vi "Available Data.vi"(8 "error in (no error)":errorcluster, 11 "Picam in":refnum<class "Picam.lvclass">) -> (0 "error out":errorcluster, 1 "Running?":bool, 2 "Data Available?":bool, 3 "Picam out":refnum<class "Picam.lvclass">)   [LabVIEW 2019, in "Picam.lvclass"]
uses:
  Picam.lvclass
  Picam.lvclass/Picam.ctl
  picam32_LabView_SDK/PICam_lib/PICam.lvlib
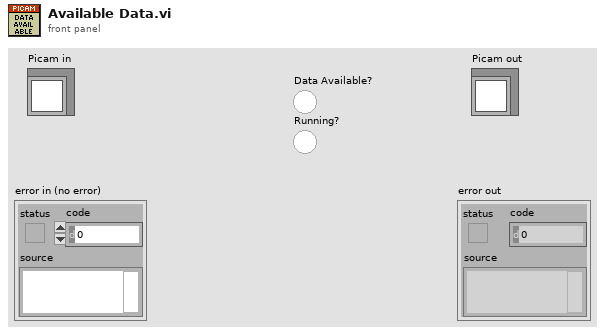
[diagram p1: front panel]
types:
  T1 = typedef "PICam.lvlib/PicamAcquisitionStatus.ctl" = cluster{"running":i32, "errors":T2, "readout_rate":dbl}
  T2 = typedef "PICam.lvlib/PicamAcquisitionErrorsMask.ctl" = enum8{"None", "DataLost", "ConnectionLost", "3", "DataNotArriving", "5", "6", "7", "ShutterOverheated", "9", "10", "11", "12", "13", "14", "15", "CameraFaulted"}
  T3 = typedef "PICam.lvlib/PicamAvailableData.ctl" = cluster{"initial_readout":u64, "readout_count":i64}
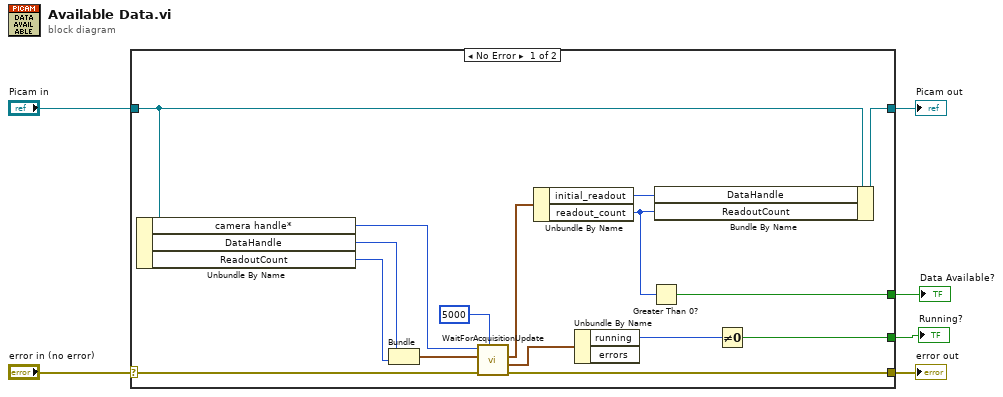
[diagram p0: block diagram]
diagram:
  n1 = case shown="No Error" "error in (no error)" {
    selector: "error in (no error)" -> [w22 w24]
    tunnel: [w20 w24] -> w5
    tunnel: [w16 w23] -> w3
    tunnel: "Picam in" -> [w21 w23]
    tunnel: [w17 _] -> w2
    tunnel: [w11 _] -> w1
    frame No Error {
      n2 = Unbundle By Name(w21) -> ("camera handle*"=w19:u64, "DataHandle"=w8:u64, "ReadoutCount"=w7:i64)
      n3 = Bundle("DataHandle"=w8, "ReadoutCount"=w7) -> (w9:cluster{"DataHandle":u64, "ReadoutCount":i64})  [unwired: 1 in]
      n4 = call "WaitForAcquisitionUpdate.vi"("piint (readout_time_out)"=i64 5000, "error in (no error)"=w22, "PicamAvailableData"=w9, "camera handle in"=w19) -> ("error out"=w20:errorcluster, "PicamAcquisitionStatus* status"=w13:T1, "PicamAvailableData* (available)"=w18:T3)  [unwired: 4 in, 1 out]
      n5 = Unbundle By Name(w18) -> ("initial_readout"=w14:u64, "readout_count"=w15:i64)
      n6 = Unbundle By Name(w13) -> ("running"=w12:i32)  [unwired: 1 out]
      n7 = Greater Than 0?(x=w15) -> (x > 0?=w17:bool)
      n8 = Bundle By Name(cluster=w21, "DataHandle"=w14, "ReadoutCount"=w15) -> (w16:refnum<class "Picam.lvclass">)
      n9 = Not Equal To 0?(x=w12) -> (x != 0?=w11:bool)
    }
    frame Error {
    }
  }
  "error out" <- w5
  "Picam out" <- w3
  "Data Available?" <- w2
  "Running?" <- w1
